vi "Test Get Debug Log Continue Refreshing.vi"(8 "error in (no error)":errorcluster, 11 "Test Case In":refnum<class "Debugger Test.lvclass">) -> (0 "error out":errorcluster, 3 "Test Case Out":refnum<class "Debugger Test.lvclass">)   [LabVIEW 2020, in "Debugger Test.lvclass"]
uses:
  Debugger Test.lvclass
  C:/Program Files (x86)/National Instruments/LabVIEW 2020/vi.lib/Astemes/LUnit/Test Case.lvclass
  source/Debugger/Debugger.lvclass
  C:/Git/astemes-triarc-debugger/source/Process/Debug Process.lvclass
  source/Debug Data/Raw Debug Data.ctl
  source/Debug Data/Debug Data.lvclass/Debug Data.ctl
  source/Process/Debug Process.lvclass/Debug Process.ctl
  <vilib>/Astemes/LUnit/Test Case.lvclass/Test Case.ctl
  01074fa8-ee8a-411d-bc8b-fc92c4f90959.vi
  <vilib>/AdvancedString/Delimited String to 1D String Array.vi
  source/Process/Public/Lifecycle/Get Lifecycle State.vi
  <vilib>/Astemes/Triarc Framework/Broadcast Event Helpers/Execution timer.vi
  source/Process/Private/SubVIs/Wait for finish.vi
  source/Process/Protected/Messaging/Enqueue Message.vi
  source/Process/Private/SubVIs/Set Lifecycle State.vi
  <vilib>/Astemes/LUnit/Palette/Pass.vi
  <vilib>/Astemes/LUnit/Palette/Fail.vi
  <vilib>/Astemes/LUnit/Compare Variants.vi
  <vilib>/Astemes/LUnit/Describe Comparison.vi
  <vilib>/Astemes/LUnit/Set Assertion Type.vi
  <vilib>/Utility/error.llb/Clear Errors.vi
  <vilib>/Astemes/LUnit/Add test result.vi
  <vilib>/Astemes/LUnit/Variant to string.vi
  <vilib>/Astemes/LUnit/LUnit Record Assertion Result.vi
  <vilib>/Astemes/LUnit/LUnit Aggregate Assertion Results.vi
  <vilib>/Astemes/LUnit/Method Result/LUnit Merge Status.vi
  <vilib>/Astemes/LUnit/LUnit Concatenate result strings.vi
  <vilib>/Utility/error.llb/Error Cluster From Error Code.vi
  <vilib>/Astemes/Triarc Framework/Broadcast Event Helpers/Dequeue Broadcast Message.vi
  <vilib>/Utility/Data Type/Get Type Information.vi
  <vilib>/Utility/LVClass/Get LV Class Name.vi
  source/Process/Debug Process.lvclass
  Debugger Test.lvclass/Debugger Test.ctl
  source/Debug Data/Debug Data.lvclass
  <vilib>/Astemes/Triarc Framework/Broadcast Event Helpers/Broadcast Event Helpers.lvlib
  C:/Git/astemes-triarc-debugger/source/Debugger/Debugger.lvclass
  C:/Git/astemes-triarc-debugger/source/Debug Data Event/Debug Data Listener.lvclass
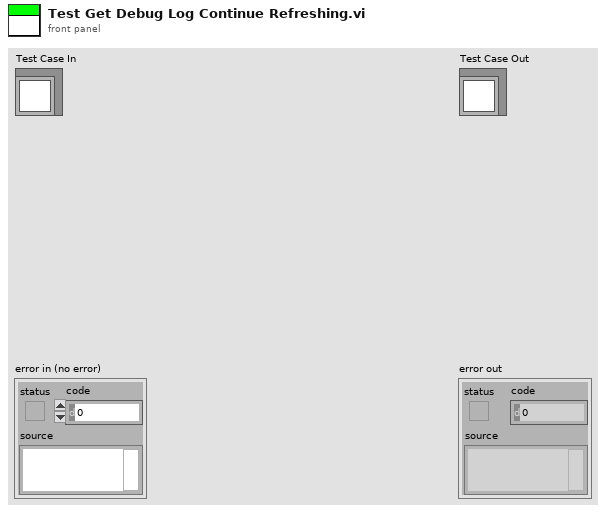
[diagram p1: front panel]
types:
  T1 = typedef "Debug Data.lvclass/Raw Debug Data.ctl" = cluster{"Action":string, "Call Chain":string, "Process":string, "Message":string, "Message Data":variant, "Time":dbl}
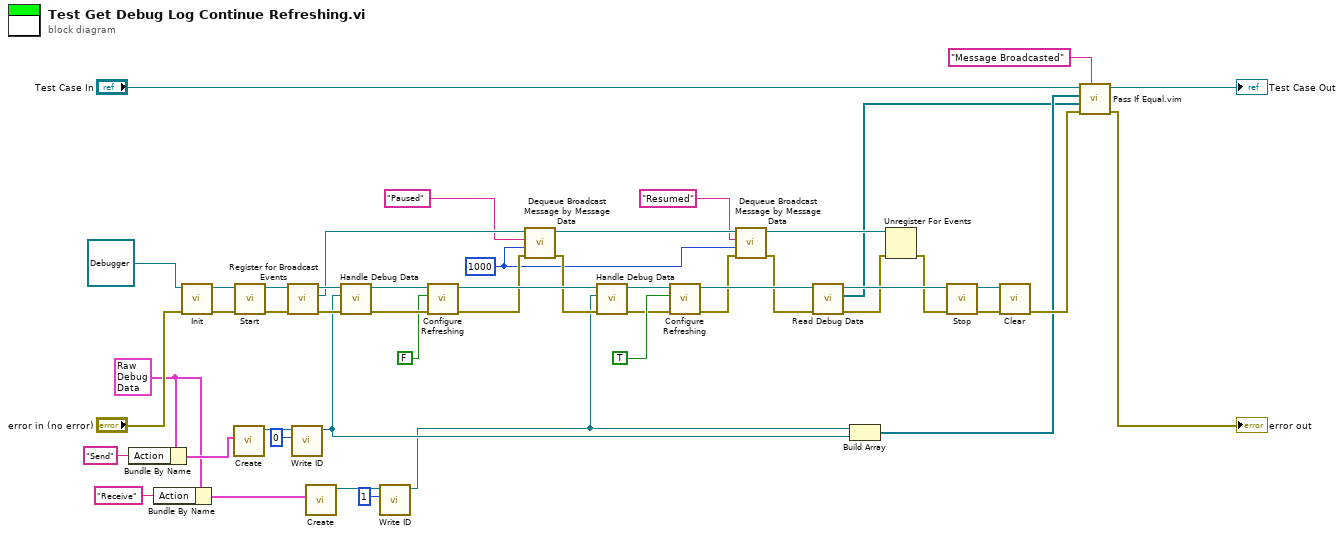
[diagram p0: block diagram]
diagram:
  w27 = T1 {"Action"="", "Call Chain"="", "Process"="", "Message"="", "Message Data"=variant, "Time"=0.0} ("Debug Data Cluster")
  w16 = 1000
  n1 = Bundle By Name(cluster=w27, "Action"="Send" ("Process")) -> (w32:T1)
  n2 = Bundle By Name(cluster=w27, "Action"="Receive" ("Process")) -> (w28:T1)
  n3 = call-dynamic "Init.vi"("error in (no error)"="error in (no error)", "Process In"=refnum<class "Debugger.lvclass"> refnum ("Debug Data Event In 2")) -> ("error out"=w45:errorcluster, "Process Out"=w46:refnum<class "Debugger.lvclass">)  [unwired: 8 in]
  n4 = call "Create.vi"("Debug Data Cluster"=w32) -> ("Debug Data out"=w6:refnum<class "Debug Data.lvclass">)  [unwired: 9 in, 1 out]
  n5 = call "Start.vi"("error in (no error)"=w45, "Process In"=w46) -> ("error out"=w43:errorcluster, "Process Out"=w44:refnum<class "Debugger.lvclass">)  [unwired: 7 in, 1 out]
  n6 = call "Register for Broadcast Events.vi"("error in (no error)"=w43, "Process In"=w44) -> ("error out"=w42:errorcluster, "Event Registration Refnum Out"=w33:refnum<event-registration>, "Process Out"=w38:refnum<class "Debugger.lvclass">)  [unwired: 7 in]
  n7 = call "Write ID.vi"("ID"=u32 0, "Debug Data in"=w6) -> ("Debug Data out"=w5:refnum<class "Debug Data.lvclass">)  [unwired: 8 in, 1 out]
  n8 = call "Create.vi"("Debug Data Cluster"=w28) -> ("Debug Data out"=w4:refnum<class "Debug Data.lvclass">)  [unwired: 9 in, 1 out]
  n9 = call-dynamic "Handle Debug Data.vi"("error in (no error)"=w42, "Debug Data.lvclass"=w5, "Debug Data Event In"=w38) -> ("error out"=w30:errorcluster, "Debug Data Event Out"=w26:refnum<class "Debugger.lvclass">)  [unwired: 7 in]
  n10 = call "Write ID.vi"("ID"=u32 1, "Debug Data in"=w4) -> ("Debug Data out"=w3:refnum<class "Debug Data.lvclass">)  [unwired: 8 in, 1 out]
  n11 = call "Configure Refreshing.vi"("error in (no error)"=w30, "Refresh?"=FALSE ("Show Send?"), "Debugger In"=w26) -> ("error out"=w20:errorcluster, "Debugger Out"=w21:refnum<class "Debugger.lvclass">)  [unwired: 7 in]
  n12 = call <vilib>:"Dequeue Broadcast Message by Message Data.vi"("error in (no error)"=w20, "Timeout (-1)"=w16, "Message Data"="Paused" ("Message"), "Event Registration Refnum"=w33) -> ("error out"=w19:errorcluster, "Event Registration Refnum Out"=w18:refnum<event-registration>)  [unwired: 3 in, 3 out]
  n13 = call-dynamic "Handle Debug Data.vi"("error in (no error)"=w19, "Debug Data.lvclass"=w3, "Debug Data Event In"=w21) -> ("error out"=w11:errorcluster, "Debug Data Event Out"=w14:refnum<class "Debugger.lvclass">)  [unwired: 7 in]
  n14 = call "Configure Refreshing.vi"("error in (no error)"=w11, "Refresh?"=TRUE, "Debugger In"=w14) -> ("error out"=w10:errorcluster, "Debugger Out"=w13:refnum<class "Debugger.lvclass">)  [unwired: 7 in]
  n15 = call <vilib>:"Dequeue Broadcast Message by Message Data.vi"("error in (no error)"=w10, "Timeout (-1)"=w16, "Message Data"="Resumed" ("Message"), "Event Registration Refnum"=w18) -> ("error out"=w9:errorcluster, "Event Registration Refnum Out"=w17:refnum<event-registration>)  [unwired: 3 in, 3 out]
  n16 = call "Read Debug Data.vi"("error in (no error)"=w9, "Debugger In"=w13) -> ("error out"=w25:errorcluster, "Data Log"=w7:refnum<class "Debug Data.lvclass">[], "Debugger Out"=w41:refnum<class "Debugger.lvclass">)  [unwired: 7 in]
  n17 = Build Array(w3, w5) -> (w8:refnum<class "Debug Data.lvclass">[])
  n18 = Unregister For Events(event registration refnum=w17, error in=w25) -> (error out=w24:errorcluster)
  n19 = call "Stop.vi"("error in (no error)"=w24, "Process In"=w41) -> ("error out"=w39:errorcluster, "Process Out"=w40:refnum<class "Debugger.lvclass">)  [unwired: 7 in, 1 out]
  n20 = call-dynamic "Clear.vi"("error in (no error)"=w39, "Process In"=w40) -> ("error out"=w35:errorcluster)  [unwired: 9 in]
  n21 = call "Pass If Equal.vim"("Description"="Message Broadcasted", "error in (no error)"=w35, "Actual"=w7, "Expected"=w8, "LUnit Test Case In"="Test Case In") -> ("error out"=→"error out":errorcluster, "LUnit Test Case Out"=→"Test Case Out":refnum<class "Debugger Test.lvclass">)  [unwired: 5 in]
